vi "ADAM_Open.vi"(10 "port":u32, 11 "VISA resource name":refnum<visa-resource-name> caption="VISA资源名称") -> (0 "错误输出":errorcluster, 3 "status":bool)   [LabVIEW 2017]
uses:
  <vilib>/Instr/_visa.llb/VISA Configure Serial Port (Instr).vi
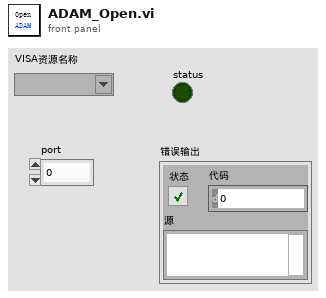
[diagram p1: front panel]
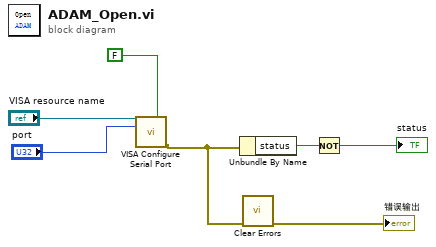
[diagram p0: block diagram]
diagram:
  n1 = call-poly "VISA Configure Serial Port"("VISA resource name"="VISA resource name", "Enable Termination\nChar (T)"=FALSE ("Enable Termination\nChar (T)"), "baud rate (9600)"="port") -> ("error out"=w3:errorcluster)  [unwired: 6 in, 6 out]
  n2 = Unbundle By Name(w3) -> ("status"=w5:bool)
  n3 = call <vilib>:"Clear Errors.vi"("error in (no error)"=w3) -> ("error out"=→"错误输出":errorcluster)  [unwired: 5 in, 1 out]
  n4 = Not(x=w5) -> (.not. x?=→"status":bool)
